vi "AA PM Main.vi"() -> ()   [LabVIEW 2024]
doc: "This template is for the Queued Message Handler design pattern.\n\nThe Event Handling Loop generates messages based on user interface actions.\n\nThe Message Handling Loop processes messages generated by the Event Handling Loop, or by other messages. The messages are string values, so new messages can be added easily to the Message Cases case structure in the Message Handling Loop. Each message cluster can also provide an optional value for Message Data, which is a variant that can be converted to whatever message-specific data is required."
uses:
  controls/AA PM UI Data.ctl
  support/Message Queue/Enqueue Message (Single).vi
  support/Message Queue/Enqueue Message (Array).vi
  <vilib>/Utility/file.llb/Read Delimited Spreadsheet (string).vi
  <vilib>/Utility/error.llb/Error Cluster From Error Code.vi
  <vilib>/ErrorRing/Error Ring.xnode
  support/Message Queue/AA PM Message Queue.lvlib
  support/User Event - Stop/AA PM User Event - Stop.lvlib
panel:
  out "st mess":string caption="Status Message"
  out "Qty found":i32 caption="Quantity found"
  out "Avg meas":dbl caption="Average measure" format="%.2f"
  in  "Stop":bool
  out "WG":dbl[][](graph)
  in  "Tol%":dbl(slide) caption="Tolerance%" min=0.0 scale=0.0..10.0
  in  "Start":bool
  in  "CSV Data File":path caption="Path"
  out "data qty":i32 caption="Data length"
  out "empty":bool caption="Empty?"
  in  "Min Thr":dbl(slide) caption="Minimal Threshold [W]" min=0.0 scale=0.0..100.0
  in  "Exit":bool
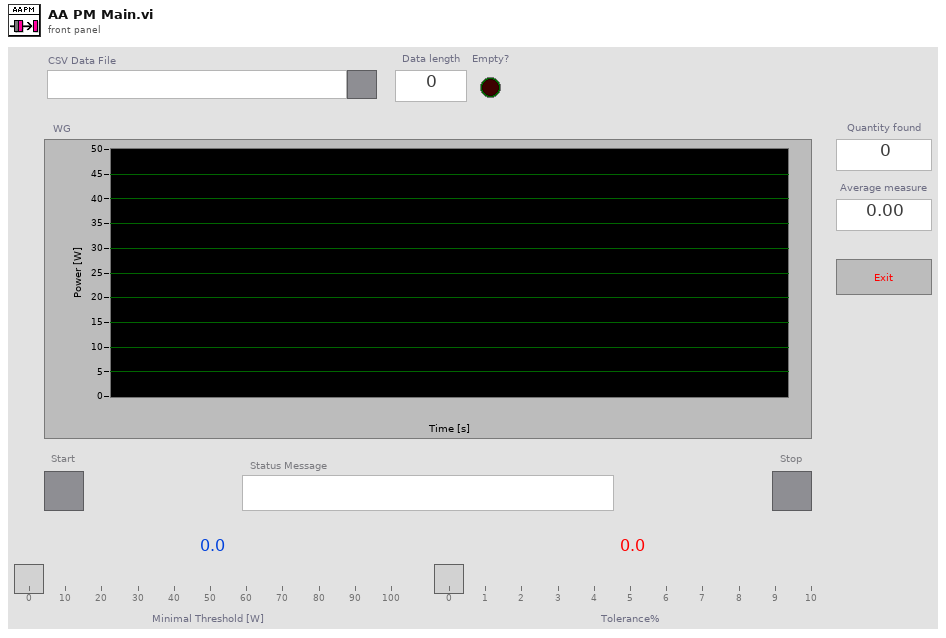
[diagram p1: front panel]
types:
  T1 = typedef "AA PM UI Data.ctl" = cluster{"empty":bool, "st mess":string, "data qty":i32, "Do Something Ref":refnum<vi>, "Do Something Else Ref":refnum<vi>, "Data Display Ref":refnum<vi>, "Exit Button Ref":refnum<vi>, "raw data":dbl[]}
  T2 = typedef "AA PM Message Queue.lvlib/All Message Queues.ctl" = cluster{"MAIN":refnum<queue>}
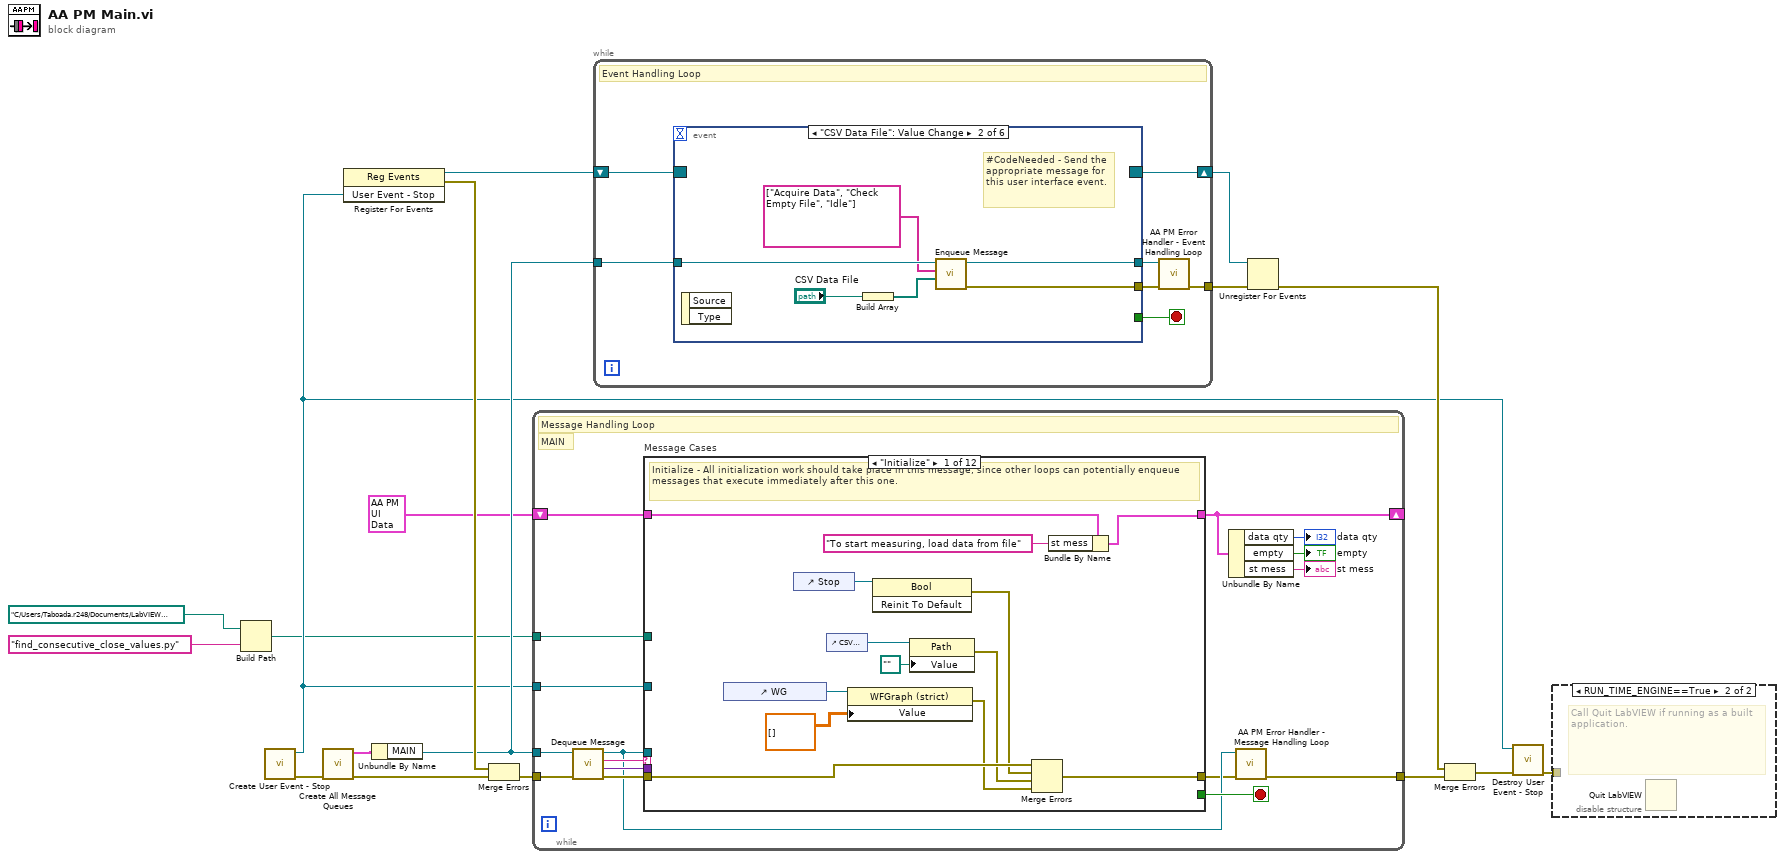
[diagram p0: block diagram]
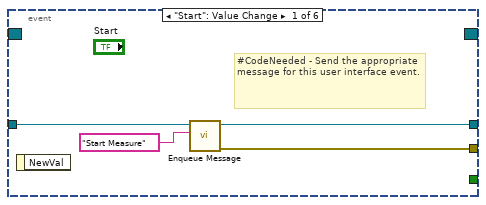
[diagram p3: hidden frame]
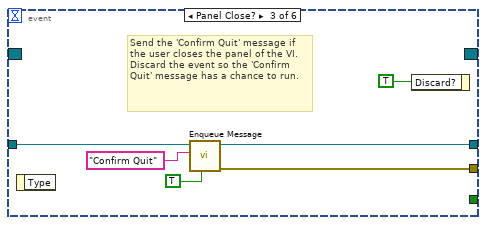
[diagram p4: hidden frame]
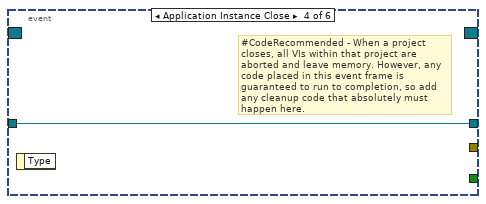
[diagram p5: hidden frame]
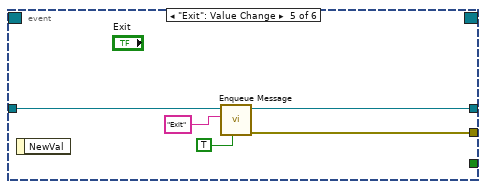
[diagram p6: hidden frame]
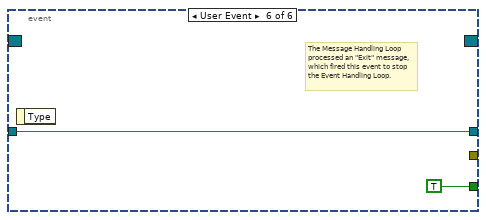
[diagram p7: hidden frame]
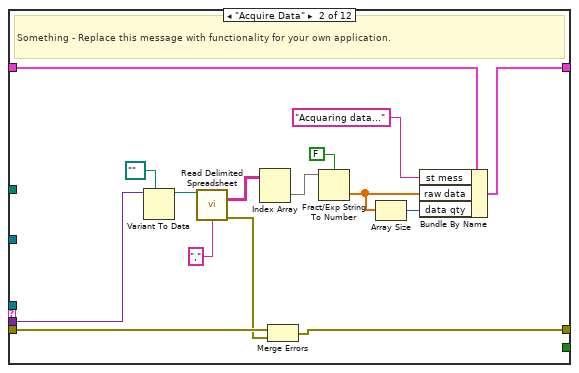
[diagram p8: hidden frame]
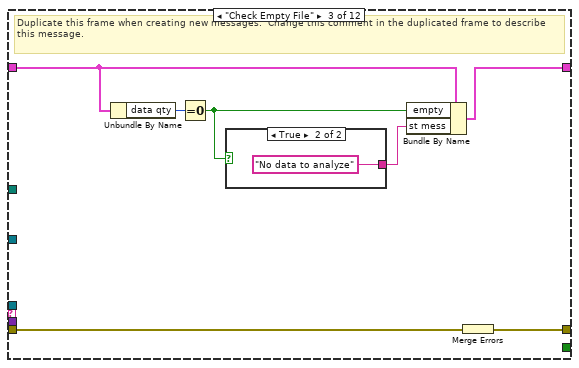
[diagram p9: hidden frame]
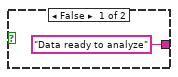
[diagram p10: hidden frame]
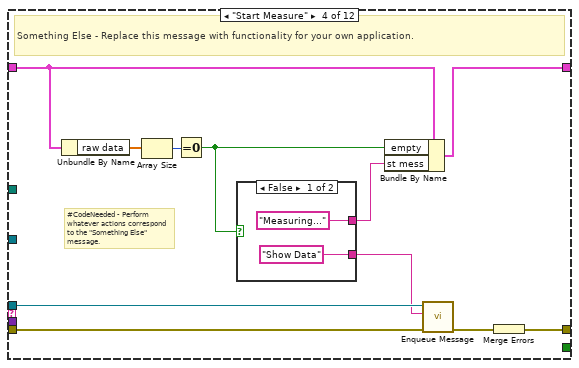
[diagram p11: hidden frame]
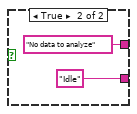
[diagram p12: hidden frame]
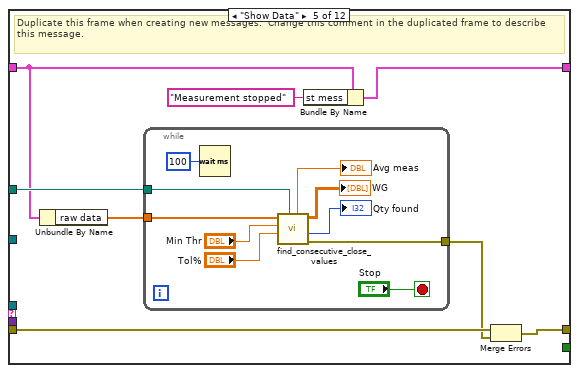
[diagram p13: hidden frame]
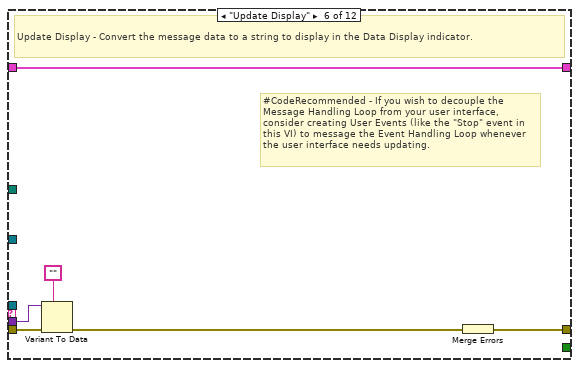
[diagram p14: hidden frame]
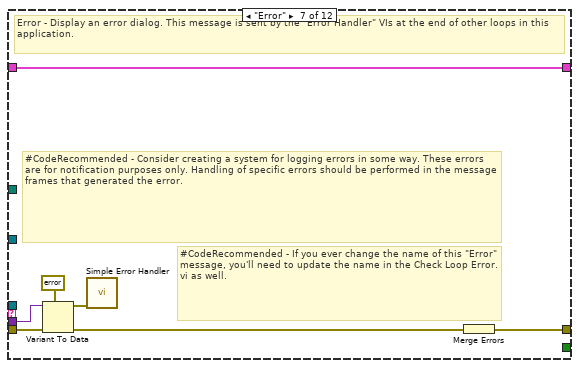
[diagram p15: hidden frame]
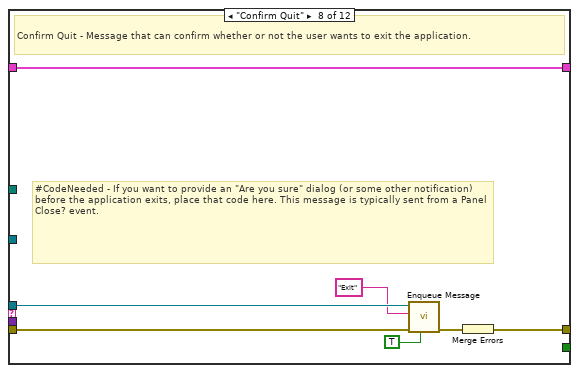
[diagram p16: hidden frame]
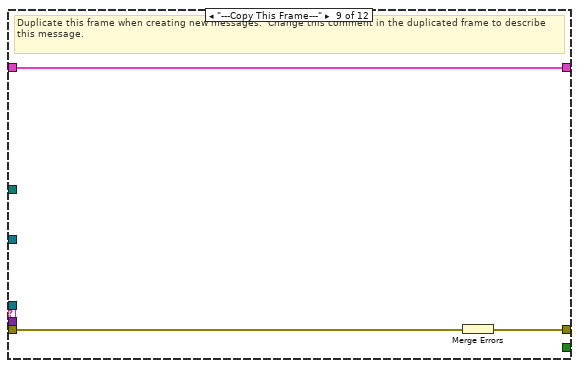
[diagram p17: hidden frame]
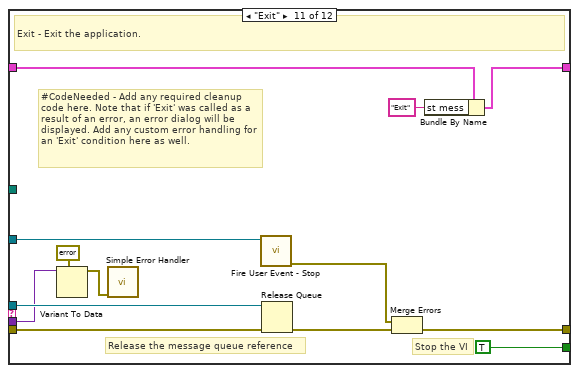
[diagram p19: hidden frame]
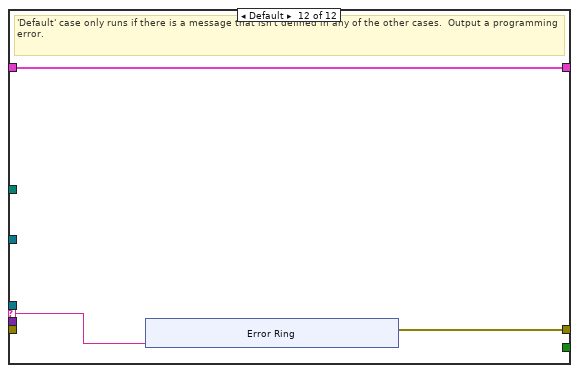
[diagram p20: hidden frame]
diagram:
  n1 = Build Path(base path=path "C:/Users/Taboada.r248/Documents/LabVIEW Projects/LabVIEW-2024-and-Python/pyhthon_modules", name or relative path="find_consecutive_close_values.py") -> (appended path=w2:path)
  n2 = call "Create User Event - Stop.vi"() -> ("error out"=w13:errorcluster, "User Event - Stop"=w5:refnum<user-event>)  [unwired: 10 in]
  n3 = call "Create All Message Queues.vi"("error in (no error)"=w13) -> ("error out"=w17:errorcluster, "Message Queues out"=w16:T2)  [unwired: 9 in]
  n4 = register-events(w5) -> (reference out=w6:refnum<event-registration>, error out=w18:errorcluster)  [unwired: 2 in]
  n5 = Unbundle By Name(w16) -> ("MAIN"=w14:refnum<queue>)
  n6 = Merge Errors(w18, w17) -> (w4:errorcluster)
  n7 = while {
    tunnel: w14 -> [w27]
    shift-right: [w23] -> _
    shift-left: T1 {"empty"=FALSE, "st mess"="", "data qty"=0, "Do Something Ref"=refnum, "Do Something Else Ref"=refnum, "Data Display Ref"=refnum, "Exit Button Ref"=refnum, "raw data"=[]} ("Data Cluster") -> [w34]
    tunnel: w5 -> [w32]
    tunnel: w4 -> [w31]
    tunnel: [w25] -> w15
    tunnel: w2 -> [w20]
    stop <- w33 stop-if-true
    # "MAIN"
    # "Message Handling Loop"
    n8 = call "Dequeue Message.vi"("error in (no error)"=w31, "Message Queue"=w27) -> ("error out"=w30:errorcluster, "Message Data"=w28:variant, "Message"=w29:string, "dup Message Queue"=w26:refnum<queue>)  [unwired: 6 in]
    n9 = case "Message Cases" shown="\"Initialize\"" w29 {
      selector: w29 -> [_ _ _ _ _ _ _ _ _ _ _ w143]
      tunnel: w26 -> [_ _ _ w79 _ _ _ w120 _ _ w142 _]
      tunnel: w30 -> [w43 w50 w69 w81 w94 w108 w117 w124 w127 w129 w136 _]
      tunnel: [w39 w62 w68 w82 w93 w109 w111 w122 w125 w129 w139 w144] -> w24
      tunnel: w34 -> [w45 w57 w66 w78 w89 w110 w116 w123 w126 w128 w132 w145]
      tunnel: [w44 w56 w65 w75 w87 w110 w116 w123 w126 w128 w131 w145] -> w23
      tunnel: [_ _ _ _ _ _ _ _ _ _ TRUE _] -> w33
      tunnel: w28 -> [_ w53 _ _ _ w107 w115 _ _ _ w133 _]
      tunnel: w32 -> [_ _ _ _ _ _ _ _ _ _ w138 _]
      tunnel: w20 -> [_ _ _ _ w91 _ _ _ _ _ _ _]
      frame "Initialize" {
        # "Initialize - All initialization work should take place in this message, since other loops can potentially enqueue messages that execute immediately after this one."
        n10 = control-ref of="WG"() -> (w47:refnum<vi>)
        n11 = control-ref of="Stop"() -> (w36:refnum<vi>)
        n12 = control-ref of="CSV Data File"() -> (w41:refnum<vi>)
        n13 = property class="WFGraph (strict)"(reference=w47, "Value"=dbl[][] []) -> (error out=w38:errorcluster)  [unwired: 1 in, 1 out]
        n14 = invoke class="Bool" method="Reinit To Default"(reference=w36) -> (error out=w35:errorcluster)  [unwired: 2 in, 2 out]
        n15 = property class="Path"(reference=w41, "Value"=path "") -> (error out=w37:errorcluster)  [unwired: 1 in, 1 out]
        n16 = Merge Errors(w43, w35, w37, w38) -> (w39:errorcluster)
        n17 = Bundle By Name(cluster=w45, "st mess"="To start measuring, load data from file" ("Initial Message")) -> (w44:T1)
      }
      frame "Acquire Data" {
        # "Something - Replace this message with functionality for your own application."
        n18 = Variant To Data(type=path "", Variant=w53) -> (data=w51:path)  [unwired: 1 in, 1 out]
        n19 = call-poly <vilib>:"Read Delimited Spreadsheet.vi"("file path (dialog if empty)"=w51, "delimiter (\\t)"=",") -> ("all rows"=w61:string[][], "error out"=w49:errorcluster)  [unwired: 8 in, 4 out]
        n20 = Index Array(array=w61) -> (element=w59:string[])  [unwired: 2 in]
        n21 = Merge Errors(w50, w49) -> (w62:errorcluster)
        n22 = Fract/Exp String To Number(use system decimal point (T)=FALSE, string=w59) -> (number=w55:dbl[])  [unwired: 2 in, 1 out]
        n23 = Array Size(array=w55) -> (size(s)=w54:i32)
        n24 = Bundle By Name(cluster=w57, "st mess"="Acquaring data...", "raw data"=w55, "data qty"=w54) -> (w56:T1)
      }
      frame "Check Empty File" {
        # "Duplicate this frame when creating new messages.  Change this comment in the duplicated frame to describe this message."
        n25 = Unbundle By Name(w66) -> ("data qty"=w67:i32)
        n26 = Equal To 0?(x=w67) -> (x = 0?=w64:bool)
        n27 = case shown="True" w64 {
          tunnel: ["Data ready to analyze" "No data to analyze"] -> w63
          frame False {
          }
          frame True {
          }
        }
        n28 = Bundle By Name(cluster=w66, "empty"=w64, "st mess"=w63) -> (w65:T1)
        n29 = Merge Errors(w69) -> (w68:errorcluster)
      }
      frame "Start Measure" {
        # "#CodeNeeded - Perform whatever actions correspond to the \"Something Else\" message."
        # "Something Else - Replace this message with functionality for your own application."
        n30 = Unbundle By Name(w78) -> ("raw data"=w77:dbl[])
        n31 = Array Size(array=w77) -> (size(s)=w76:i32)
        n32 = Equal To 0?(x=w76) -> (x = 0?=w74:bool)
        n33 = case shown="False" w74 {
          tunnel: ["Show Data" "Idle" ("Message")] -> w73
          tunnel: ["Measuring..." "No data to analyze"] -> w72
          frame False {
          }
          frame True {
          }
        }
        n34 = Bundle By Name(cluster=w78, "empty"=w74, "st mess"=w72) -> (w75:T1)
        n35 = call-poly "Enqueue Message.vi"("error in (no error)"=w81, "Message"=w73, "Message Queue"=w79) -> ("error out"=w80:errorcluster)  [unwired: 7 in, 1 out]
        n36 = Merge Errors(w80) -> (w82:errorcluster)
      }
      frame "Show Data" {
        # "Duplicate this frame when creating new messages.  Change this comment in the duplicated frame to describe this message."
        n37 = Unbundle By Name(w89) -> ("raw data"=w92:dbl[])
        n38 = while {
          tunnel: w92 -> [w104]
          tunnel: w91 -> [w102]
          tunnel: [w99] -> w90
          stop <- "Stop" stop-if-true
          n39 = Wait (ms)(milliseconds to wait=u32 100) -> ()  [unwired: 1 out]
          n40 = call "find_consecutive_close_values.vi"("module path"=w102, "tolerance"="Tol%", "min_threshold"="Min Thr", "data"=w104) -> ("error out"=w99:errorcluster, "#_elements_found"=→"Qty found":i32, "Measures"=→"WG":dbl[][], "average"=→"Avg meas":dbl)  [unwired: 2 in, 2 out]
        }
        n41 = Bundle By Name(cluster=w89, "st mess"="Measurement stopped") -> (w87:T1)
        n42 = Merge Errors(w94, w90) -> (w93:errorcluster)
      }
      frame "Update Display" {
        # "#CodeRecommended - If you wish to decouple the Message Handling Loop from your user interface, consider creating User Events (like the \"Stop\" event in this VI) to message the Event Handling Loop whenever the user interface needs updating."
        # "Update Display - Convert the message data to a string to display in the Data Display indicator."
        n43 = Variant To Data(error in=w108, type="", Variant=w107) -> (error out=w105:errorcluster)  [unwired: 1 out]
        n44 = Merge Errors(w105) -> (w109:errorcluster)
      }
      frame "Error" {
        # "#CodeRecommended - If you ever change the name of this \"Error\" message, you'll need to update the name in the Check Loop Error.vi as well."
        # "#CodeRecommended - Consider creating a system for logging errors in some way. These errors are for notification purposes only. Handling of specific errors should be performed in the message frames that generated the error."
        # "Error - Display an error dialog. This message is sent by the \"Error Handler\" VIs at the end of other loops in this application."
        n45 = Variant To Data(error in=w117, type=errorcluster {"status"=FALSE, "code"=0, "source"=""} ("error constant"), Variant=w115) -> (data=w113:errorcluster, error out=w112:errorcluster)
        n46 = call <vilib>:"Simple Error Handler.vi"("error in (no error)"=w113) -> ()  [unwired: 4 in, 5 out]
        n47 = Merge Errors(w112) -> (w111:errorcluster)
      }
      frame "Confirm Quit" {
        # "#CodeNeeded - If you want to provide an \"Are you sure\" dialog (or some other notification) before the application exits, place that code here. This message is typically sent from a Panel Close? event."
        # "Confirm Quit - Message that can confirm whether or not the user wants to exit the application."
        n48 = call-poly "Enqueue Message.vi"("Priority Message? (F)"=TRUE, "error in (no error)"=w124, "Message"="Exit", "Message Queue"=w120) -> ("error out"=w121:errorcluster)  [unwired: 6 in, 1 out]
        n49 = Merge Errors(w121) -> (w122:errorcluster)
      }
      frame "---Copy This Frame---" {
        # "Duplicate this frame when creating new messages.  Change this comment in the duplicated frame to describe this message."
        n50 = Merge Errors(w127) -> (w125:errorcluster)
      }
      frame "Idle" {
      }
      frame "Exit" {
        # "Stop the VI"
        # "Release the message queue reference"
        # "#CodeNeeded - Add any required cleanup code here. Note that if 'Exit' was called as a result of an error, an error dialog will be displayed. Add any custom error handling for an 'Exit' condition here as well."
        # "Exit - Exit the application."
        n51 = Variant To Data(type=errorcluster {"status"=FALSE, "code"=0, "source"=""} ("error constant"), Variant=w133) -> (data=w134:errorcluster)  [unwired: 1 in, 1 out]
        n52 = call <vilib>:"Simple Error Handler.vi"("error in (no error)"=w134) -> ()  [unwired: 4 in, 5 out]
        n53 = call "Fire User Event - Stop.vi"("User Event - Stop"=w138) -> ("error out"=w137:errorcluster)  [unwired: 10 in]
        n54 = Release Queue(queue=w142, error in (no error)=w136) -> (error out=w140:errorcluster)  [unwired: 1 in, 2 out]
        n55 = Merge Errors(w137, w140) -> (w139:errorcluster)
        n56 = Bundle By Name(cluster=w132, "st mess"="Exit") -> (w131:T1)
      }
      frame Default {
        # "'Default' case only runs if there is a message that isn't defined in any of the other cases.  Output a programming error."
        n57 = xnode "Error Ring"("parameter 0"=w143) -> ("error out"=w144:errorcluster)
      }
    }
    n58 = Unbundle By Name(w23) -> ("data qty"=→"data qty":i32, "empty"=→"empty":bool, "st mess"=→"st mess":string)
    n59 = call "AA PM Error Handler - Message Handling Loop.vi"("error in (no error)"=w24, "Message Queue"=w26) -> ("dup error in"=w25:errorcluster)  [unwired: 8 in, 1 out]
  }
  n60 = while {
    tunnel: w14 -> [w159]
    shift-right: [w157] -> w10
    shift-left: w6 -> [w158]
    tunnel: [w153] -> w7
    stop <- w155 stop-if-true
    # "Event Handling Loop"
    n61 = event shown="[1] \"CSV Data File\": Value Change" {
      selector: w158 -> [_ _ _ _ _ _]
      dyn-events: [_ _ _ _ _ _] -> w157
      timeout: _ -> [_ _ _ _ _ _]
      tunnel: [_ _ _ _ _ TRUE ("Discard?")] -> w155
      tunnel: w159 -> [w163 w169 w174 w176 w181 w183]
      tunnel: [w160 w167 w173 _ w180 _] -> w156
      tunnel: [w162 w168 w172 w176 w179 w183] -> w154
      event "Start": Value Change {
        # "#CodeNeeded - Send the appropriate message for this user interface event."
        n62 = event-data() -> ()  [unwired: 1 in, 1 out]
        n63 = call-poly "Enqueue Message.vi"("Message"="Start Measure", "Message Queue"=w163) -> ("error out"=w160:errorcluster, "dup Message Queue"=w162:refnum<queue>)  [unwired: 8 in]
      }
      event "CSV Data File": Value Change {
        # "#CodeNeeded - Send the appropriate message for this user interface event."
        n64 = event-data() -> ()  [unwired: 1 in, 2 out]
        n65 = Build Array("CSV Data File") -> (w164:path[])
        n66 = call-poly "Enqueue Message.vi"("Message Data Array"=w164, "Message Array"=string[] ["Acquire Data", "Check Empty File", "Idle"], "Message Queue"=w169) -> ("error out"=w167:errorcluster, "dup Message Queue"=w168:refnum<queue>)  [unwired: 7 in]
      }
      event Panel Close? {
        # "Send the 'Confirm Quit' message if the user closes the panel of the VI. Discard the event so the 'Confirm Quit' message has a chance to run."
        n67 = event-data() -> ()  [unwired: 1 in, 1 out]
        n68 = call-poly "Enqueue Message.vi"("Priority Message? (F)"=TRUE, "Message"="Confirm Quit", "Message Queue"=w174) -> ("error out"=w173:errorcluster, "dup Message Queue"=w172:refnum<queue>)  [unwired: 7 in]
        n69 = event-data("Discard?"=TRUE) -> ()  [unwired: 1 in, 1 out]
      }
      event Application Instance Close {
        # "#CodeRecommended - When a project closes, all VIs within that project are aborted and leave memory. However, any code placed in this event frame is guaranteed to run to completion, so add any cleanup code that absolutely must happen here."
        n70 = event-data() -> ()  [unwired: 1 in, 1 out]
      }
      event "Exit": Value Change {
        n71 = event-data() -> ()  [unwired: 1 in, 1 out]
        n72 = call-poly "Enqueue Message.vi"("Priority Message? (F)"=TRUE, "Message"="Exit", "Message Queue"=w181) -> ("error out"=w180:errorcluster, "dup Message Queue"=w179:refnum<queue>)  [unwired: 7 in]
      }
      event User Event {
        # "The Message Handling Loop processed an \"Exit\" message, which fired this event to stop the Event Handling Loop."
        n73 = event-data() -> ()  [unwired: 1 in, 1 out]
      }
    }
    n74 = call "AA PM Error Handler - Event Handling Loop.vi"("error in (no error)"=w156, "Message Queue"=w154) -> ("dup error in"=w153:errorcluster)  [unwired: 8 in, 1 out]
  }
  n75 = Unregister For Events(event registration refnum=w10, error in=w7) -> (error out=w11:errorcluster)
  n76 = Merge Errors(w11, w15) -> (w12:errorcluster)
  n77 = call "Destroy User Event - Stop.vi"("error in (no error)"=w12, "User Event - Stop"=w5) -> ("error out"=w8:errorcluster)  [unwired: 9 in]
  n78 = disable-structure shown="RUN_TIME_ENGINE==True" {
    disable-tunnel: w8 -> [_ _]
    frame condition #0 (active) {
    }
    frame condition #1 {
      # "Call Quit LabVIEW if running as a built application."
      n79 = Quit LabVIEW() -> ()  [unwired: 1 in]
    }
  }
